vi "Set Ramp Rate.vi"(8 "error in (no error)":errorcluster, 11 "79XRP in":refnum<class "79XRP.lvclass">) -> (0 "error out":errorcluster, 3 "79XRP out":refnum<class "79XRP.lvclass">)   [LabVIEW 2019, in "79XRP.lvlib" / "79XRP.lvclass"]
uses:
  Library/79XRP.lvclass
  C:/Users/Public/Documents/Development/builds/Instruments/PowerSupply.lvlibp/Library/PowerSupply.lvclass
  Accessors/Read Local Resource.vi
  Accessors/Write Local Resource.vi
  <instrlib>/Keysight RP7900 Series/Keysight RP7900 Series.lvlib
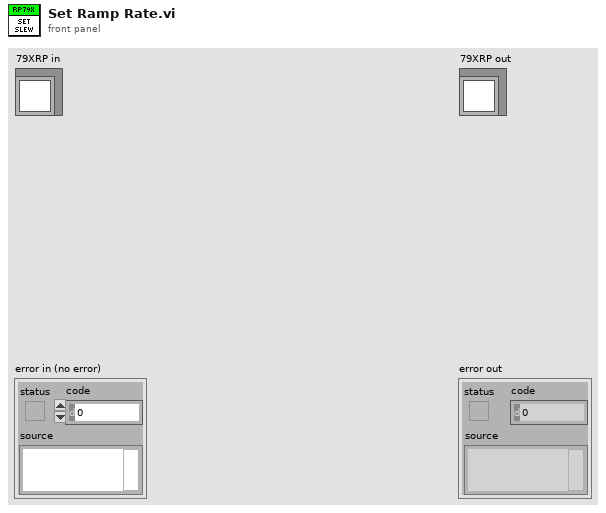
[diagram p1: front panel]
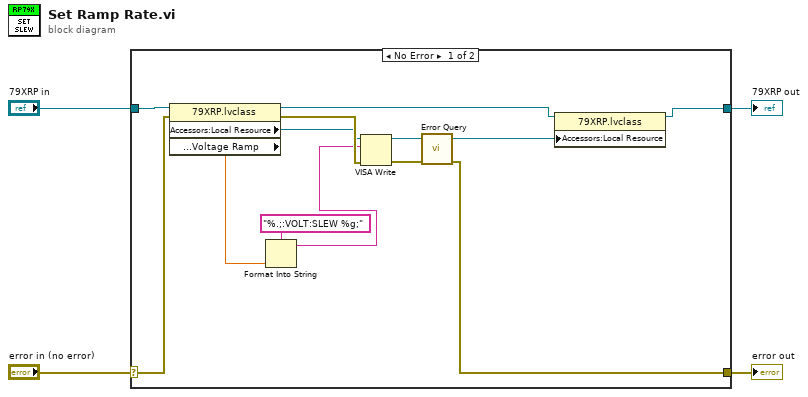
[diagram p0: block diagram]
diagram:
  n1 = case shown="No Error" "error in (no error)" {
    selector: "error in (no error)" -> [w16 w19]
    tunnel: [w8 w19] -> w3
    tunnel: [w6 w18] -> w1
    tunnel: "79XRP in" -> [w17 w18]
    frame No Error {
      n2 = property class="79XRP.lvclass"(reference=w17, error in=w16) -> (reference out=w5:refnum<class "79XRP.lvclass">, error out=w13:errorcluster, "Accessors:Local Resource"=w12:refnum<visa-resource-name>, "Accessors:Setting:Ramp:Voltage Ramp"=w10:dbl)
      n3 = Format Into String(format string="%.;:VOLT:SLEW %g;", w10) -> (resulting string=w11:string)  [unwired: 2 in, 1 out]
      n4 = VISA Write(VISA resource name=w12, write buffer=w11, error in (no error)=w13) -> (VISA resource name out=w9:refnum<visa-resource-name>, error out=w14:errorcluster)  [unwired: 1 out]
      n5 = call <instrlib>:"Error Query.vi"("error in (no error)"=w14, "VISA resource name"=w9) -> ("error out"=w8:errorcluster, "VISA resource name out"=w7:refnum<visa-resource-name>)  [unwired: 6 in, 2 out]
      n6 = property class="79XRP.lvclass"(reference=w5, "Accessors:Local Resource"=w7) -> (reference out=w6:refnum<class "79XRP.lvclass">)  [unwired: 1 in, 1 out]
    }
    frame Error {
    }
  }
  "error out" <- w3
  "79XRP out" <- w1
